vi "Logger.vi"(8 "error in":errorcluster, 9 "string":string, 10 "Function":string) -> (0 "error out":errorcluster)   [LabVIEW 2014]
panel:
  in  "base path":path
  in  "FileOpen":bool
  out "refnum out":refnum<file>
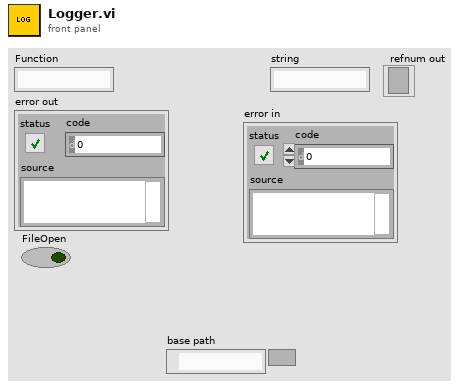
[diagram p1: front panel]
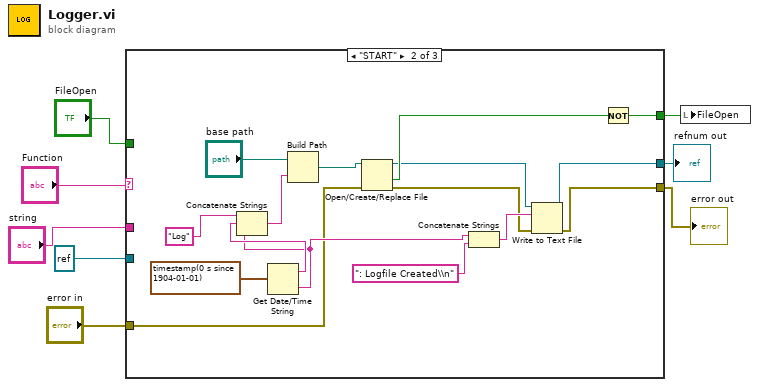
[diagram p0: block diagram]
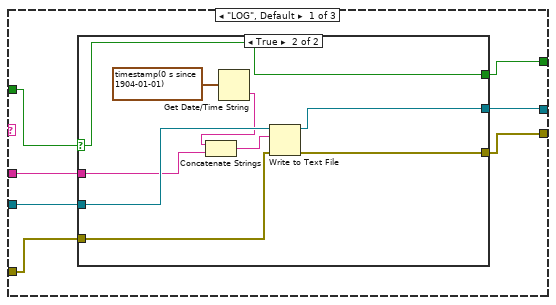
[diagram p2: hidden frame]
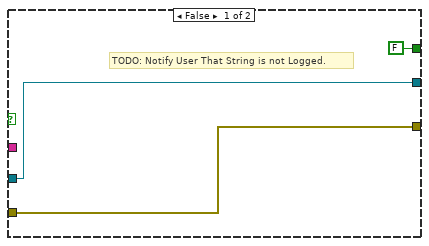
[diagram p3: hidden frame]
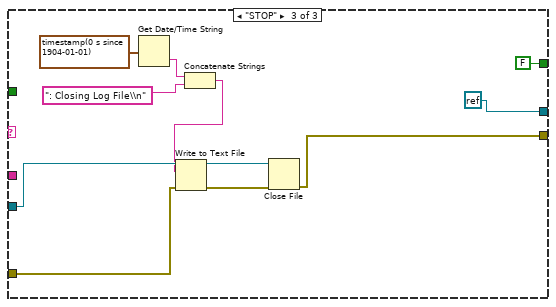
[diagram p4: hidden frame]
diagram:
  n1 = case shown="\"START\"" "Function" {
    tunnel: [w14 w30 refnum<k0> refnum] -> w7
    tunnel: [w11 w31 w48] -> w6
    tunnel: [w9 w37 FALSE] -> w4
    tunnel: "FileOpen" -> [w15 _ _]
    tunnel: refnum<file> refnum ("refnum out 2") -> [w13 _ w51]
    tunnel: "error in" -> [w12 w29 w50]
    tunnel: "string" -> [w10 _ _]
    frame "LOG", Default {
      n2 = case shown="True" w15 {
        selector: w15 -> [_ w19]
        tunnel: [w17 w27] -> w14
        tunnel: w13 -> [w17 w26]
        tunnel: w12 -> [w16 w25]
        tunnel: [w16 w24] -> w11
        tunnel: w10 -> [_ w20]
        tunnel: [FALSE w19] -> w9
        frame False {
          # "TODO: Notify User That String is not Logged."
        }
        frame True {
          n3 = Get Date/Time String(seconds (now)=timestamp(0 s since 1904-01-01)) -> (time string=w21:string)  [unwired: 2 in, 1 out]
          n4 = Concatenate Strings(w21, w20) -> (w22:string)
          n5 = Write to Text File(file (use dialog)=w26, text=w22, error in=w25) -> (refnum out=w27:refnum<file>, error out=w24:errorcluster)  [unwired: 1 in, 1 out]
        }
      }
    }
    frame "START" {
      n6 = Get Date/Time String(seconds (now)=timestamp(0 s since 1904-01-01)) -> (date string=w40:string, time string=w35:string)  [unwired: 2 in]
      n7 = Concatenate Strings("Log", w40, w35) -> (w39:string)
      n8 = Build Path(base path="base path", name or relative path=w39) -> (appended path=w43:path)
      n9 = Open/Create/Replace File(file path (use dialog)=w43, error in=w29) -> (refnum out=w34:refnum<file>, cancelled=w38:bool, error out=w32:errorcluster)  [unwired: 4 in]
      n10 = Concatenate Strings(w35, ": Logfile Created\\n") -> (w33:string)
      n11 = Write to Text File(file (use dialog)=w34, text=w33, error in=w32) -> (refnum out=w30:refnum<file>, error out=w31:errorcluster)  [unwired: 1 in, 1 out]
      n12 = Not(x=w38) -> (.not. x?=w37:bool)
    }
    frame "STOP" {
      n13 = Get Date/Time String(seconds (now)=timestamp(0 s since 1904-01-01)) -> (time string=w52:string)  [unwired: 2 in, 1 out]
      n14 = Concatenate Strings(w52, ": Closing Log File\\n") -> (w45:string)
      n15 = Write to Text File(file (use dialog)=w51, text=w45, error in=w50) -> (refnum out=w46:refnum<file>, error out=w49:errorcluster)  [unwired: 1 in, 1 out]
      n16 = Close File(refnum=w46, error in=w49) -> (error out=w48:errorcluster)  [unwired: 1 out]
    }
  }
  "refnum out" <- w7
  "error out" <- w6
  n17 = local write "FileOpen"(w4) -> ()
